vi "TCP接收测试.vi"() -> ()   [LabVIEW 2016]
panel:
  in  "停止按钮":bool
  out "error out":errorcluster
  out "接收数据":string
  in  "5s 超时":i32=5000
  in  "输入簇":cluster{"IP":string, "Port":u16}
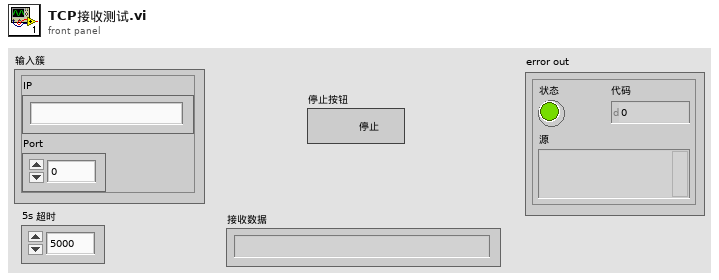
[diagram p1: front panel]
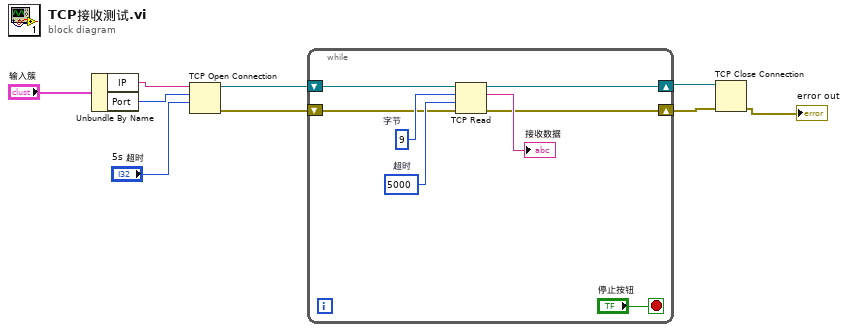
[diagram p0: block diagram]
diagram:
  n1 = Unbundle By Name("输入簇") -> ("IP"=w8:string, "Port"=w9:u16)
  n2 = TCP Open Connection(address=w8, remote port or service name=w9, timeout ms (60000)="5s 超时") -> (connection ID=w5:refnum<k5>, error out=w4:errorcluster)  [unwired: 2 in]
  n3 = while {
    shift-right: [w11] -> w3
    shift-left: w4 -> [w13]
    shift-right: [w12] -> w2
    shift-left: w5 -> [w14]
    stop <- "停止按钮" stop-if-true
    w16 = 5000  # 超时
    w15 = 9  # 字节
    n4 = TCP Read(connection ID=w14, bytes to read=w15, error in (no error)=w13, 9:w16) -> (connection ID out=w12:refnum<k5>, data out=→"接收数据":string, error out=w11:errorcluster)  [unwired: 1 in]
  }
  n5 = TCP Close Connection(connection ID=w2, error in (no error)=w3) -> (error out=→"error out":errorcluster)  [unwired: 1 in, 1 out]
